vi "Script gRPC.vi"(8 "error in":errorcluster, 10 "Generated Library Name":string, 11 "proto File Path":path) -> (0 "error out":errorcluster)   [LabVIEW 2021, in "TemplateCoreUtilities.lvlib"]
uses:
  TemplateCoreUtilities.lvlib
  <vilib>/CIF Foundation/CIF Core/CIFUtilities/CIFConfigurationFile/CIF Configuration File.lvlib
  <vilib>/CIF Foundation/CIF Core/CIFUtilities/CIFConfigurationFile/typedef/Location Type.ctl
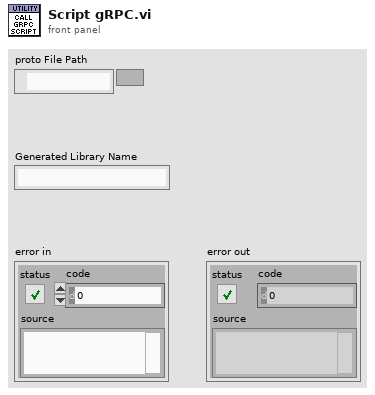
[diagram p1: front panel]
types:
  T1 = typedef "CIF Configuration File.lvlib/Location Type.ctl" = enum16{"Config File", "Manager", "Protos", "Plugins", "UI Plugins", "Logs", "Orchestrations"}
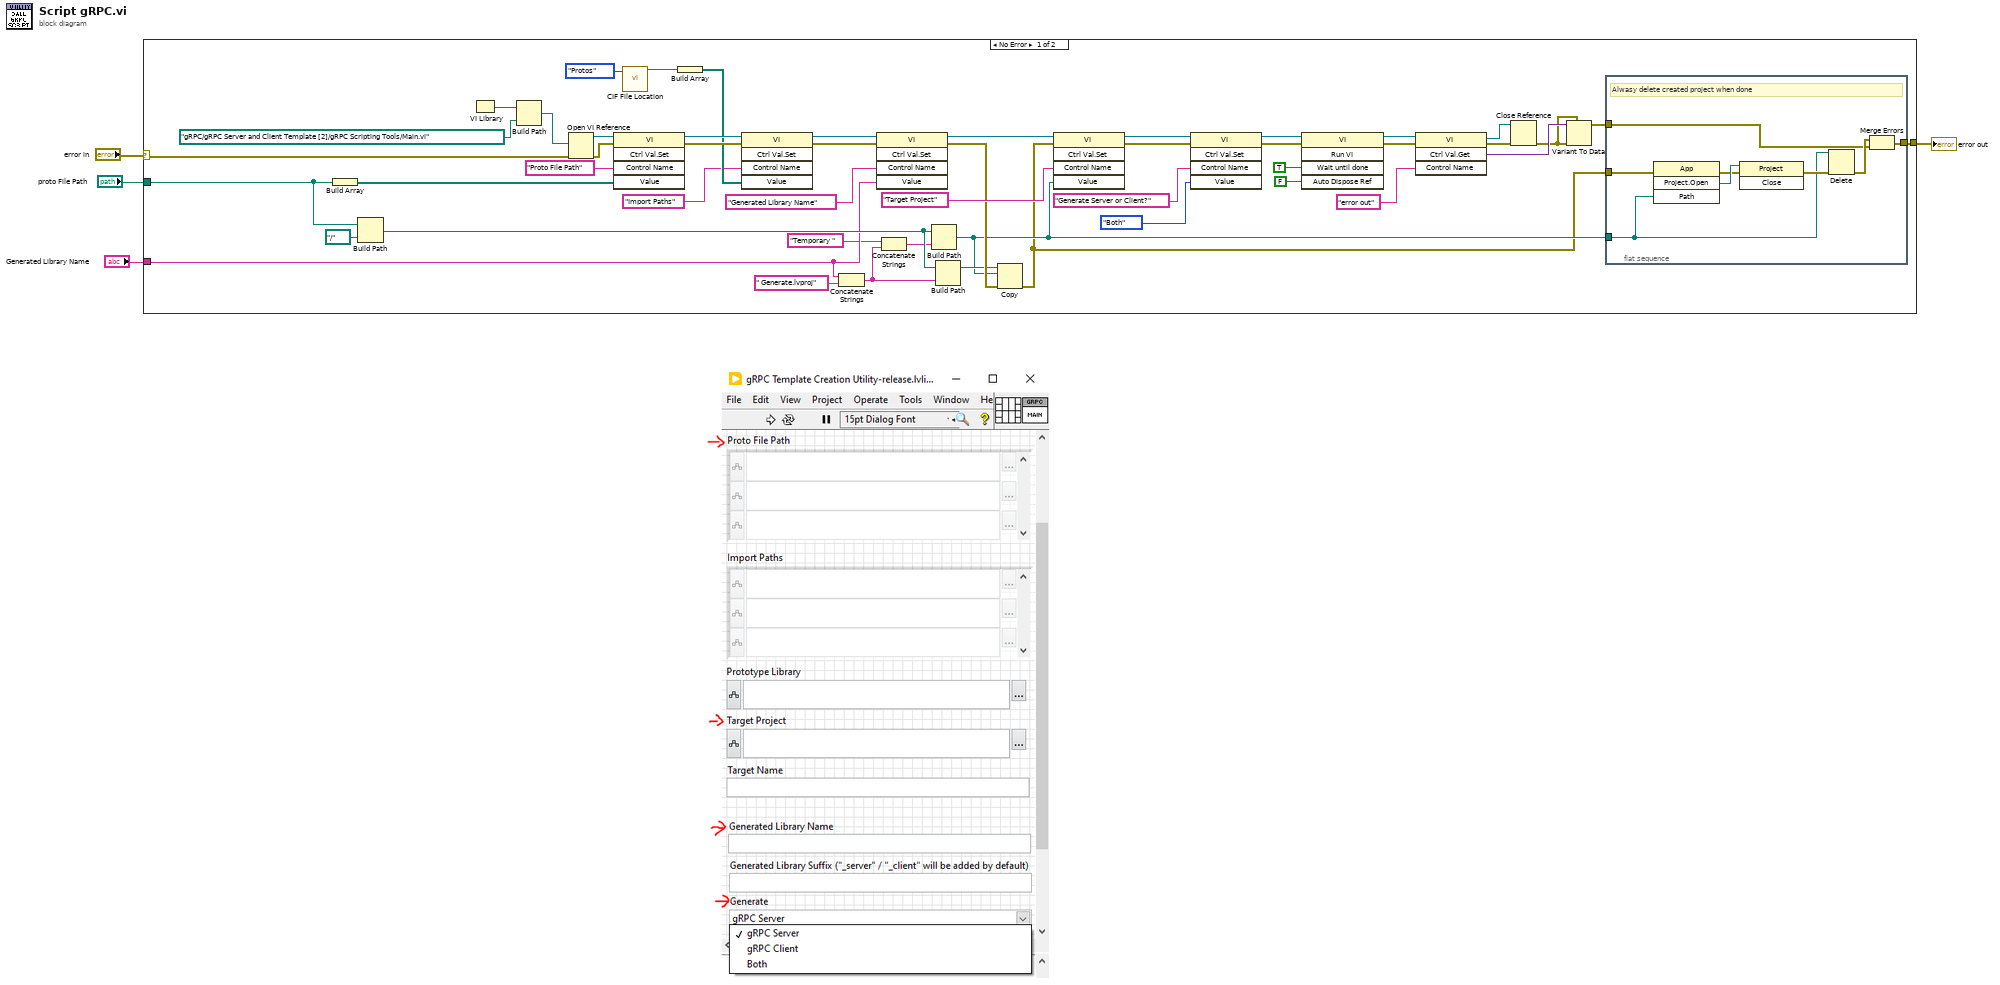
[diagram p0: block diagram]
diagram:
  n1 = case shown="No Error" "error in" {
    selector: "error in" -> [w30 w61]
    tunnel: [w12 w61] -> w4
    tunnel: "proto File Path" -> [w34 _]
    tunnel: "Generated Library Name" -> [w23 _]
    frame No Error {
      n2 = Build Array(w34) -> (w37:path[])
      n3 = Build Path(base path=w34, name or relative path=path "../..") -> (appended path=w32:path)
      n4 = VI Library() -> (path=w52:path)
      n5 = Build Path(base path=w52, name or relative path=path "gRPC/gRPC Server and Client Template [2]/gRPC Scripting Tools/Main.vi") -> (appended path=w50:path)
      n6 = Open VI Reference(vi path=w50, error in (no error)=w30) -> (vi reference=w39:refnum<vi>, error out=w38:errorcluster)  [unwired: 4 in]
      n7 = invoke class="VI" method="Ctrl Val.Set"(reference=w39, error in=w38, "Control Name"="Proto File Path", "Value"=w37) -> (reference out=w29:refnum<vi>, error out=w28:errorcluster)  [unwired: 1 in, 3 out]
      n8 = call <vilib>:"CIF File Location.vi"("LocationType"=Location_Type."Protos") -> ("Location"=w5:path)  [unwired: 10 in]
      n9 = Build Array(w5) -> (w25:path[])
      n10 = invoke class="VI" method="Ctrl Val.Set"(reference=w29, error in=w28, "Control Name"="Import Paths", "Value"=w25) -> (reference out=w27:refnum<vi>, error out=w26:errorcluster)  [unwired: 1 in, 3 out]
      n11 = Concatenate Strings(w23, " Generate.lvproj" ("string")) -> (w21:string)
      n12 = invoke class="VI" method="Ctrl Val.Set"(reference=w27, error in=w26, "Control Name"="Generated Library Name", "Value"=w23) -> (reference out=w47:refnum<vi>, error out=w31:errorcluster)  [unwired: 1 in, 3 out]
      n13 = Concatenate Strings("Temporary " ("string"), w21) -> (w18:string)
      n14 = Build Path(base path=w32, name or relative path=w18) -> (appended path=w19:path)
      n15 = Build Path(base path=w32, name or relative path=w21) -> (appended path=w20:path)
      n16 = Copy(8:w31, 10:w19, 11:w20) -> (0:w7:errorcluster)  [unwired: 2 in, 2 out]
      n17 = invoke class="VI" method="Ctrl Val.Set"(reference=w47, error in=w7, "Control Name"="Target Project", "Value"=w19) -> (reference out=w45:refnum<vi>, error out=w44:errorcluster)  [unwired: 1 in, 3 out]
      n18 = invoke class="VI" method="Ctrl Val.Set"(reference=w45, error in=w44, "Control Name"="Generate Server or Client?", "Value"=enum16{"gRPC Server", "gRPC Client", "Both"}."Both" ("Generate")) -> (reference out=w41:refnum<vi>, error out=w40:errorcluster)  [unwired: 1 in, 3 out]
      n19 = invoke class="VI" method="Run VI"(reference=w41, error in=w40, "Wait until done"=TRUE ("Wait Until Done"), "Auto Dispose Ref"=FALSE ("Auto Dispose Reference")) -> (reference out=w16:refnum<vi>, error out=w17:errorcluster)  [unwired: 1 in, 3 out]
      n20 = invoke class="VI" method="Ctrl Val.Get"(reference=w16, error in=w17, "Control Name"="error out") -> (reference out=w9:refnum<vi>, error out=w10:errorcluster, "Get Control Value Variant"=w14:variant)  [unwired: 1 in, 1 out]
      n21 = Close Reference(reference=w9, error in (no error)=w10) -> (error out=w8:errorcluster)
      n22 = Variant To Data(error in=w8, type=w8, Variant=w14) -> (data=w13:errorcluster)  [unwired: 1 out]
      n23 = flat-sequence {
        tunnel: w19 -> [w57]
        tunnel: w13 -> [w55]
        tunnel: [w54] -> w12
        tunnel: w7 -> [w53]
        frame #0 {
          # "Alwasy delete created project when done"
          n24 = invoke class="App" method="Project.Open"(error in=w53, "Path"=w57) -> (error out=w59:errorcluster, "Project:Open"=w60:refnum<vi>)  [unwired: 2 in, 2 out]
          n25 = invoke class="Project" method="Close"(reference=w60, error in=w59) -> (error out=w58:errorcluster)  [unwired: 1 in, 2 out]
          n26 = Delete(path (use dialog)=w57, error in=w58) -> (error out=w56:errorcluster)  [unwired: 3 in, 2 out]
          n27 = Merge Errors(w56, w55) -> (w54:errorcluster)
        }
      }
    }
    frame Error {
    }
  }
  "error out" <- w4
